vi "Update.vi"(8 "error in (no error)":errorcluster, 10 "Message in":refnum<class "UpdateMessage.lvclass">, 11 "ImageStack in":refnum<class "ImageStack.lvclass">) -> (0 "error out":errorcluster, 3 "ImageStack out":refnum<class "ImageStack.lvclass">)   [LabVIEW 2012, in "ImageStack.lvclass"]
doc: "The update method processes the command 'update'. \n\nThe command 'update' is used for receiving new values to be set to the private data of the class. This could be seen as a public set method for setting new parameters to the private class data."
uses:
  ImageStack.lvclass
  <vilib>/Distrio/Murmex/UpdateMessage/UpdateMessage.lvclass
  ImageStack.lvclass/ImageStack.ctl
  <vilib>/Distrio/Murmex/Murmex/Murmex.lvclass
panel:
  # "This method is called when the UPDATE\ntrigger is sent. \n\nOverride this method when your component needs to\nrespond to this trigger. \n\nCall parent for proper implementation"
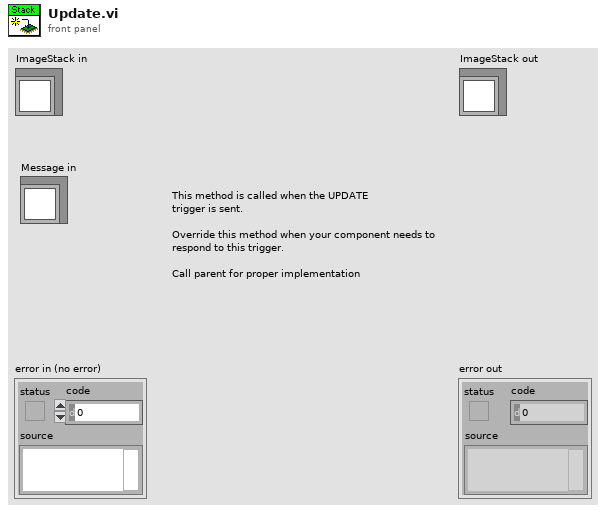
[diagram p1: front panel]
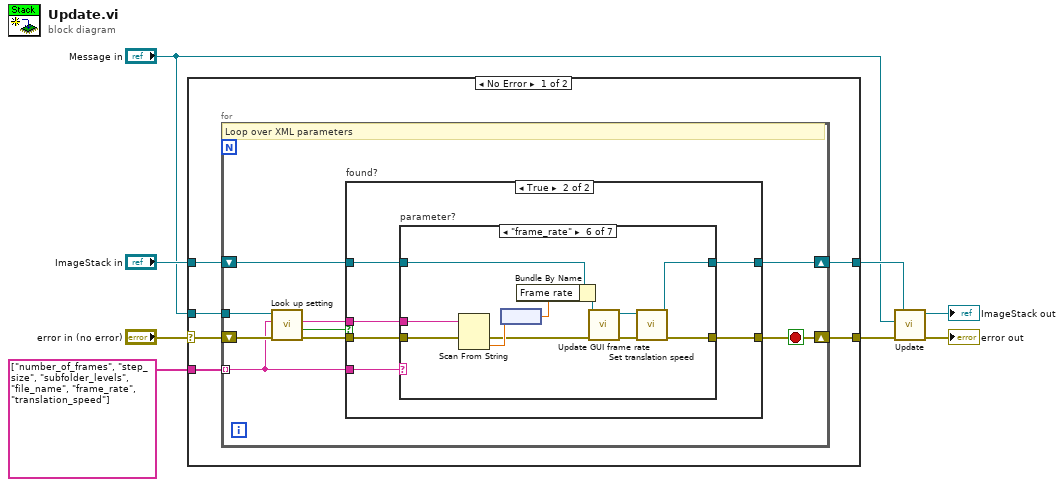
[diagram p0: block diagram]
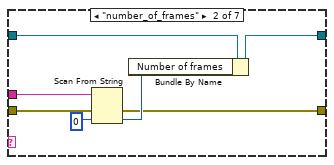
[diagram p4: hidden frame]
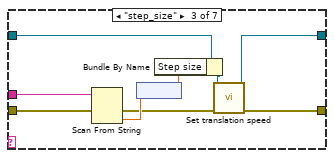
[diagram p5: hidden frame]
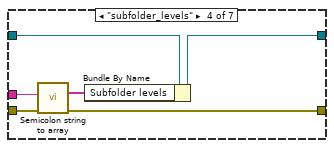
[diagram p6: hidden frame]
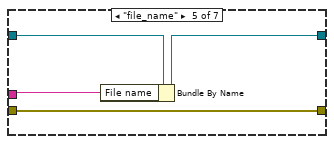
[diagram p7: hidden frame]
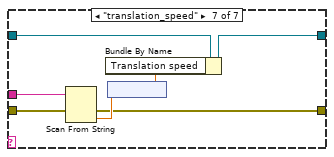
[diagram p8: hidden frame]
diagram:
  n1 = case shown="No Error" "error in (no error)" {
    selector: "error in (no error)" -> [w14 w79]
    tunnel: [w9 w79] -> w1
    tunnel: [w12 w78] -> w6
    tunnel: "ImageStack in" -> [w13 w78]
    tunnel: "Message in" -> [w11 _]
    tunnel: string[] ["number_of_frames", "step_size", "subfolder_levels", "file_name", "frame_rate", "translation_speed"] -> [w10 _]
    frame No Error {
      n2 = for {
        shift-right: [w15] -> w9
        shift-left: w14 -> [w22]
        shift-right: [w16] -> w12
        shift-left: w13 -> [w18]
        tunnel: w11 -> [w23]
        tunnel: w10 -> [w17] mode=indexing
        stop <- w15 stop-if-true
        # "Loop over XML parameters"
        n3 = call <vilib>:"Look up setting.vi"("error in (no error)"=w22, "tag name"=w17, "UpdateMessage in"=w23) -> ("error out"=w20:errorcluster, "found?"=w21:bool, "value"=w19:string)  [unwired: 5 in, 1 out]
        n4 = case "found?" shown="True" w21 {
          tunnel: w20 -> [w24 w29]
          tunnel: w19 -> [_ w30]
          tunnel: w18 -> [w25 w28]
          tunnel: w17 -> [_ w31]
          tunnel: [w24 w27] -> w15
          tunnel: [w25 w26] -> w16
          frame False {
          }
          frame True {
            n5 = case "parameter?" shown="\"frame_rate\"" w31 {
              tunnel: w30 -> [_ w40 w49 w53 w56 w64 w72]
              tunnel: w29 -> [w32 w39 w48 w52 w57 w70 w75]
              tunnel: w28 -> [w33 w37 w47 w55 w59 w66 w73]
              tunnel: [w32 w35 w42 w51 w57 w69 w74] -> w27
              tunnel: [w33 w34 w41 w54 w58 w65 w71] -> w26
              frame Default {
              }
              frame "number_of_frames" {
                n6 = Scan From String(input string=w40, error in=w39, default 1=u16 0) -> (error out=w35:errorcluster, output 1=w36:u16)  [unwired: 2 in, 2 out]
                n7 = Bundle By Name(cluster=w37, "Number of frames"=w36) -> (w34:refnum<class "ImageStack.lvclass">)
              }
              frame "step_size" {
                n8 = Scan From String(input string=w49, error in=w48) -> (error out=w43:errorcluster, output 1=w46:dbl)  [unwired: 3 in, 2 out]
                n9 = node(w46) -> (w45:dbl[unit])
                n10 = Bundle By Name(cluster=w47, "Step size"=w45) -> (w44:refnum<class "ImageStack.lvclass">)
                n11 = call-dynamic "Set translation speed.vi"("error in (no error)"=w43, "ImageStack in"=w44) -> ("error out"=w42:errorcluster, "ImageStack out"=w41:refnum<class "ImageStack.lvclass">)  [unwired: 8 in]
              }
              frame "subfolder_levels" {
                n12 = call "Semicolon string to array.vi"("error in"=w52, "Semicolon string"=w53) -> ("error out"=w51:errorcluster, "String array"=w50:string[])  [unwired: 8 in]
                n13 = Bundle By Name(cluster=w55, "Subfolder levels"=w50) -> (w54:refnum<class "ImageStack.lvclass">)
              }
              frame "file_name" {
                n14 = Bundle By Name(cluster=w59, "File name"=w56) -> (w58:refnum<class "ImageStack.lvclass">)
              }
              frame "frame_rate" {
                n15 = Scan From String(input string=w64, error in=w70) -> (error out=w63:errorcluster, output 1=w67:dbl)  [unwired: 3 in, 2 out]
                n16 = node(w67) -> (w68:dbl[unit])
                n17 = Bundle By Name(cluster=w66, "Frame rate"=w68) -> (w61:refnum<class "ImageStack.lvclass">)
                n18 = call-dynamic "Update GUI frame rate.vi"("error in (no error)"=w63, "ImageStack in"=w61) -> ("error out"=w62:errorcluster, "ImageStack out"=w60:refnum<class "ImageStack.lvclass">)  [unwired: 8 in]
                n19 = call-dynamic "Set translation speed.vi"("error in (no error)"=w62, "ImageStack in"=w60) -> ("error out"=w69:errorcluster, "ImageStack out"=w65:refnum<class "ImageStack.lvclass">)  [unwired: 8 in]
              }
              frame "translation_speed" {
                n20 = Scan From String(input string=w72, error in=w75) -> (error out=w74:errorcluster, output 1=w76:dbl)  [unwired: 3 in, 2 out]
                n21 = node(w76) -> (w77:dbl[unit])
                n22 = Bundle By Name(cluster=w73, "Translation speed"=w77) -> (w71:refnum<class "ImageStack.lvclass">)
              }
            }
          }
        }
      }
    }
    frame Error {
    }
  }
  n23 = call-parent "Update.vi"("error in (no error)"=w1, "Message in"="Message in", "Murmex in"=w6) -> ("error out"=→"error out":errorcluster, "Murmex out"=→"ImageStack out":refnum<class "ImageStack.lvclass">)  [unwired: 7 in]
